vi "Connected.vi"(8 "error in (no error)":errorcluster, 11 "input in":refnum<class "input.lvclass">) -> (0 "error out":errorcluster, 2 "connected":bool, 3 "input out":refnum<class "input.lvclass">)   [LabVIEW 2015, in "input.lvclass"]
uses:
  input.lvclass
  input.lvclass/input.ctl
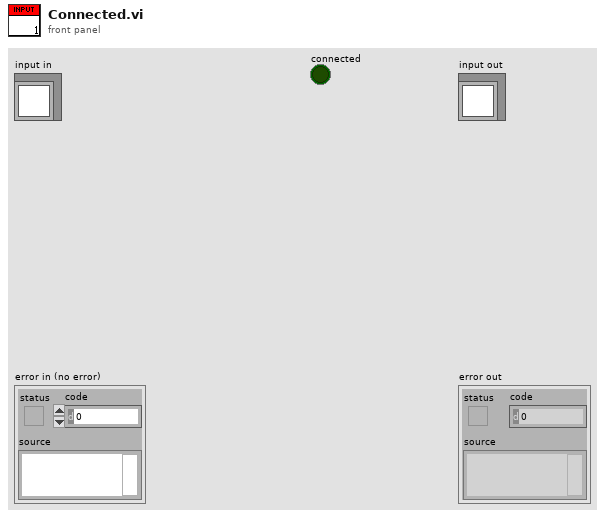
[diagram p1: front panel]
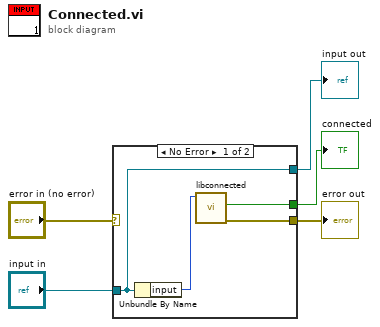
[diagram p0: block diagram]
diagram:
  n1 = case shown="No Error" "error in (no error)" {
    selector: "error in (no error)" -> [_ w11]
    tunnel: [w9 w11] -> w4
    tunnel: [w6 w10] -> w2
    tunnel: "input in" -> [w6 w10]
    tunnel: [w8 _] -> w1
    frame No Error {
      n2 = Unbundle By Name(w6) -> ("input"=w7:i32)
      n3 = call "libconnected.vi"("input"=w7) -> ("error out"=w9:errorcluster, "connected"=w8:bool)  [unwired: 9 in]
    }
    frame Error {
    }
  }
  "error out" <- w4
  "input out" <- w2
  "connected" <- w1
